vi "Bundle Script_Named (Un)Bundler Remove Unwired.vi"(8 "error in":errorcluster, 11 "Affected Items":T1) -> (0 "error out":errorcluster, 2 "Objects":refnum<vi>[](array[refnum]))   [LabVIEW 2023]
uses:
  top/BundleMagic.ctl
panel:
  out "Unwired Indicies":i32[](array[numeric])
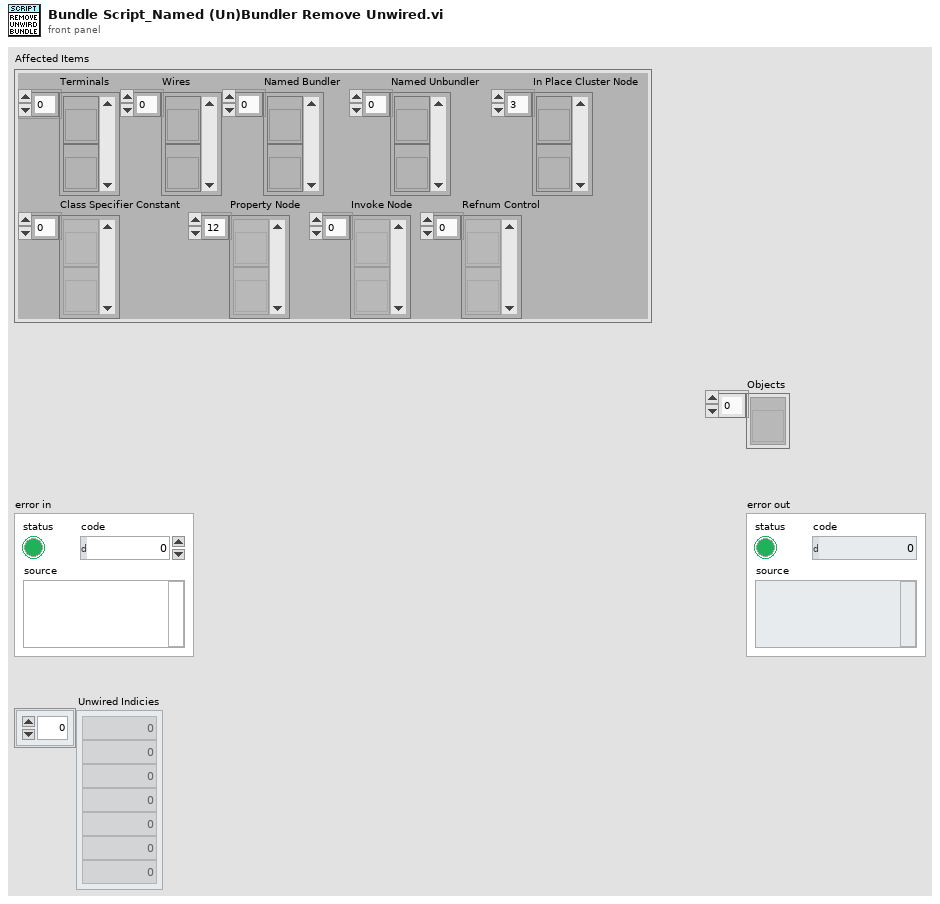
[diagram p1: front panel]
types:
  T1 = typedef "BundleMagic.ctl" = cluster{"Terminals":refnum<vi>[], "Wires":refnum<vi>[], "Named Bundler":refnum<vi>[], "Named Unbundler":refnum<vi>[], "In Place Cluster Node":refnum<vi>[], "Class Specifier Constant":refnum<vi>[], "Property Node":refnum<vi>[], "Invoke Node":refnum<vi>[], "Refnum Control":refnum<vi>[]}
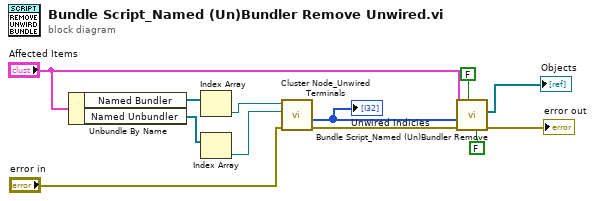
[diagram p0: block diagram]
diagram:
  n1 = Unbundle By Name("Affected Items") -> ("Named Bundler"=w9:refnum<vi>[], "Named Unbundler"=w8:refnum<vi>[])
  n2 = Index Array(array=w9) -> (element=w7:refnum<vi>)  [unwired: 1 in]
  n3 = Index Array(array=w8) -> (element=w6:refnum<vi>)  [unwired: 1 in]
  n4 = call "Cluster Node_Unwired Terminals.vi"("error in"="error in", "Named Unbundler Ref"=w6, "Named Bundler Ref"=w7) -> ("error out"=w4:errorcluster, "Unwired Indices For Removal"=w5:i32[])  [unwired: 6 in, 1 out]
  "Unwired Indicies" <- w5
  n5 = call "Bundle Script_Named (Un)Bundler Remove.vi"("Hide Full Names"=FALSE ("Change Full Name Visibilty Status"), "Change Full Name Visibilty Status"=FALSE, "error in"=w4, "Selected Item Indices"=w5, "Affected Items"="Affected Items") -> ("error out"=→"error out":errorcluster, "Objects"=→"Objects":refnum<vi>[])  [unwired: 5 in]
